vi "HK Channel Write Channel Configuration File.vi"(8 "error in (no error)":errorcluster, 10 "Channel Configuration File":path, 11 "HK Channel in":refnum<class "HK Table.lvclass">) -> (0 "error out":errorcluster, 3 "HK Channel out":refnum<class "HK Table.lvclass">)   [LabVIEW 2019, in "HK Table.lvclass"]
uses:
  HK Table.lvclass
  HK Table.lvclass/HK Table.ctl
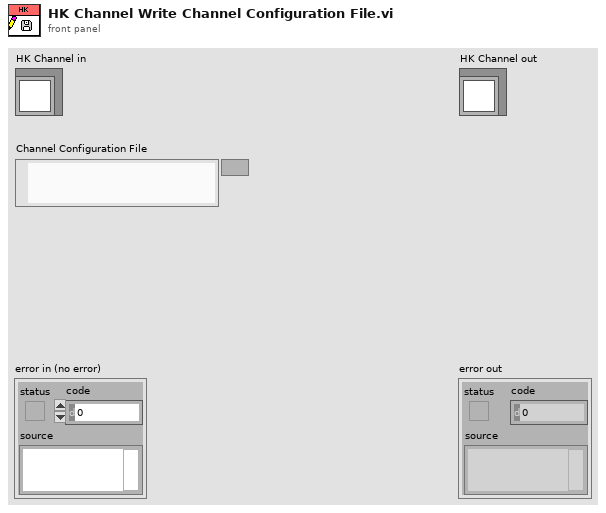
[diagram p1: front panel]
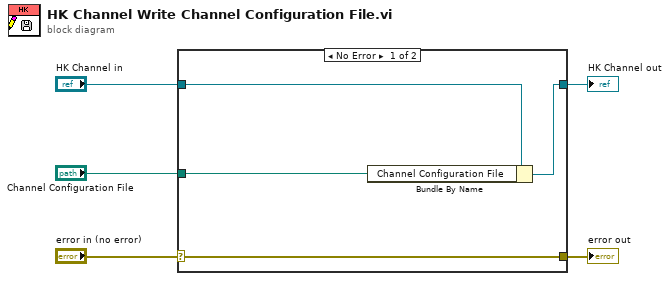
[diagram p0: block diagram]
diagram:
  n1 = case shown="No Error" "error in (no error)" {
    selector: "error in (no error)" -> [w9 w10]
    tunnel: [w9 w10] -> w4
    tunnel: [w7 w11] -> w2
    tunnel: "HK Channel in" -> [w8 w11]
    tunnel: "Channel Configuration File" -> [w6 _]
    frame No Error {
      n2 = Bundle By Name(cluster=w8, "Channel Configuration File"=w6) -> (w7:refnum<class "HK Table.lvclass">)
    }
    frame Error {
    }
  }
  "error out" <- w4
  "HK Channel out" <- w2
